vi "Build.vi"(8 "error in (no error)":errorcluster, 9 "build":bool, 11 "AB_UI_Fmwrk_Build in":refnum<class "AB_UI_Frmwk_Build.lvclass">) -> (0 "error out":errorcluster, 3 "AB_UI_Fmwrk_Build out":refnum<class "AB_UI_Frmwk_Build.lvclass">)   [LabVIEW 2020, in "AB_UI_Frmwk_Build.lvclass"]
uses:
  <vilib>/AppBuilder/AB_Classes/Build/UI/AB_UI_Frmwk_Build.lvclass
  <resource>/Framework/Providers/Builds/AppBuilder/SRdB/AB_SRdB_Action.ctl
  <vilib>/AppBuilder/AB_Classes/Build/AB_Build.lvclass
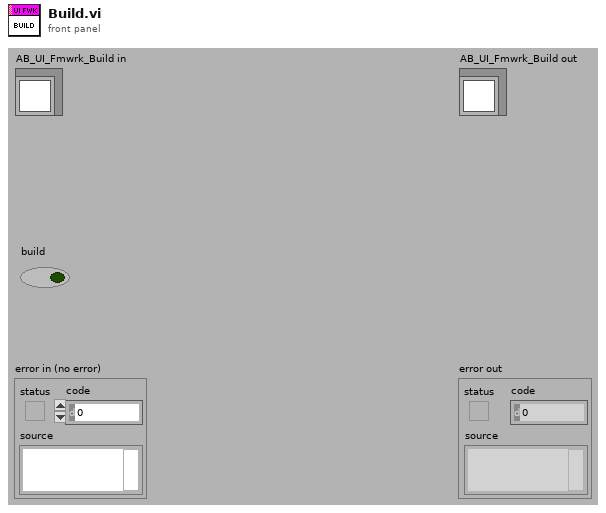
[diagram p1: front panel]
types:
  T1 = typedef "AB_SRdB_Action.ctl" = enum16{"read", "write", "create", "delete", "initialize", "unInitialize", "getLock", "readAll", "writeAll"}
  T2 = typedef "AB_Build.ctl" = cluster{"buildSpecName":string, "buildSpecDescription":string, "destinations":refnum<class "AB_Destination.lvclass">[], "exclusionOption":T3, "defaultLanguage":string, "supportedLanguages":string[], "excludedDirectories":path[], "buildContext":refnum<vi>, "buildObject":T4, "preview":bool, "programatic":bool, "progressBarEvents":T5, "userLog_Path":path, "preActionID":string, "preAction_Path":path, "postActionID":string, "postAction_Path":path, "eng_checkForBrokenVIs?":bool, "eng_verboseLinkerErrors?":bool, "localDest_Path":path, "targetDest_Path":path, "removeVIObject":u16, "cache":refnum<class "PreviewCache.lvclass">, "use cache":bool, "previewCache_ID":string, "buildCache_ID":string, "eng_TempLocalDest_Path":path, "eng_collectDependencies?":bool, "versionInfo":cluster{"buildVersion":cluster{"major":u16, "minor":u16, "patch":u16, "build":u16}, "autoIncrement":bool}, "eng_enableVIChecksums":bool}
  T3 = typedef "AB_Exclusion_Option.ctl" = cluster{"typedefs":bool, "polymorphicVIs":bool, "unusedLibraryItems":bool, "modifyLibraryFile":bool, "edit-timeDependencies":bool, "inlineVIs":bool, "dependent PPLs":bool, "dependent DLLs":bool}
  T4 = typedef "ItemRef.ctl" = u64
  T5 = typedef "provcom_ProgressBar_Events.ctl" = cluster{"newJob":refnum<user-event>, "newItem":refnum<user-event>, "errorMsg":T6, "cancel":refnum<user-event>}
  T6 = typedef "mxLvBuildError.ctl" = refnum<user-event>
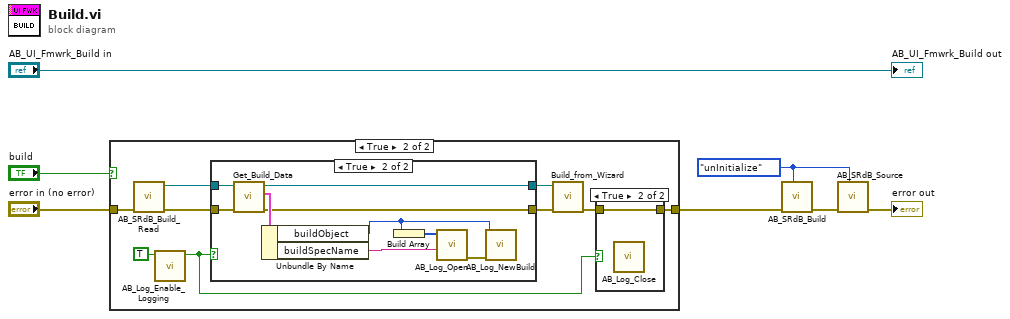
[diagram p0: block diagram]
diagram:
  w5 = AB_SRdB_Action."unInitialize" ("action")
  n1 = case shown="True" "build" {
    tunnel: "error in (no error)" -> [w8 w13]
    tunnel: [w8 w16] -> w6
    frame False {
    }
    frame True {
      n2 = call <resource>:"AB_SRdB_Build_Read.vi"("error in (no error)"=w13) -> ("error out"=w11:errorcluster, "build out"=w12:refnum<class "AB_Build.lvclass">)  [unwired: 9 out]
      n3 = call <vilib>:"AB_Log_Enable_Logging.vi"("read INI"=TRUE) -> ("log?"=w14:bool)  [unwired: 1 in, 9 out]
      n4 = case shown="True" w14 {
        tunnel: [w21 w24] -> w17
        tunnel: w11 -> [w21 w26]
        tunnel: w12 -> [w20 w27]
        tunnel: [w20 w25] -> w10
        frame False {
        }
        frame True {
          n5 = call <vilib>:"Get_Build_Data.vi"("error in (no error)"=w26, "Class in"=w27) -> ("error out"=w24:errorcluster, "data"=w28:T2, "Class out"=w25:refnum<class "AB_Build.lvclass">)  [unwired: 7 out]
          n6 = Unbundle By Name(w28) -> ("buildObject"=w22:T4, "buildSpecName"=w23:string)
          n7 = Build Array(w22) -> (w29:T4[])
          n8 = call <vilib>:"AB_Log_Open.vi"("build spec name"=w23, "Objects"=w29) -> ("error out"=w30:errorcluster)  [unwired: 1 in, 8 out]
          n9 = call <vilib>:"AB_Log_NewBuild.vi"("error in (no error)"=w30, "Object"=w22) -> ()  [unwired: 10 out]
        }
      }
      n10 = call-dynamic "Build_from_Wizard.vi"("error in (no error)"=w17, "AB_Build in"=w10) -> ("error out"=w15:errorcluster)  [unwired: 2 in, 7 out]
      n11 = case shown="True" w14 {
        tunnel: [w18 w19] -> w16
        tunnel: w15 -> [w18 w19]
        frame False {
        }
        frame True {
          n12 = call <vilib>:"AB_Log_Close.vi"() -> ()  [unwired: 1 in, 11 out]
        }
      }
    }
  }
  n13 = call <resource>:"AB_SRdB_Build.vi"("action"=w5, "error in (no error)"=w6) -> ("error out"=w4:errorcluster)  [unwired: 1 in, 8 out]
  n14 = call <resource>:"AB_SRdB_Source.vi"("action"=w5, "error in (no error)"=w4) -> ("error out"=→"error out":errorcluster)  [unwired: 3 in, 6 out]
  "AB_UI_Fmwrk_Build out" <- "AB_UI_Fmwrk_Build in"
